vi "Convert error to warning.vi"(1 "Codes":i32[](array[numeric]), 5 "error in":errorcluster) -> (19 "error out":errorcluster)   [LabVIEW 2020]
doc: "If \"code\" is one of the code numbers given in \"Codes\", resets error status to \"no error\" and adds \"Warning: \" to \"source\"."
panel:
  # "If \"code\" is one of the code numbers given in \"Codes\", resets\nerror status to \"no error\" and adds \"Warning: \" to \"source\"."
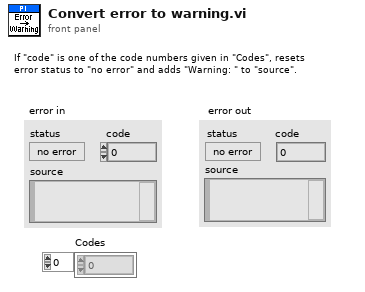
[diagram p1: front panel]
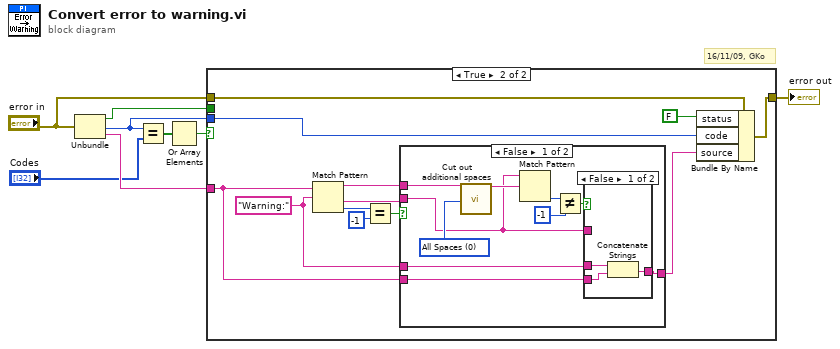
[diagram p0: block diagram]
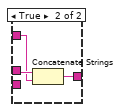
[diagram p3: hidden frame]
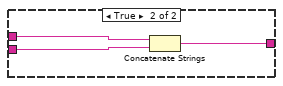
[diagram p4: hidden frame]
diagram:
  # "16/11/09, GKo"
  n1 = Unbundle("error in") -> ("status"=w7:bool, "code"=w5:i32, "source"=w6:string)
  n2 = Equal?(x=w5, y="Codes") -> (x = y?=w2:bool[])
  n3 = Or Array Elements(Boolean array=w2) -> (logical OR=w1:bool)
  n4 = case shown="True" w1 {
    tunnel: "error in" -> [w9 w21]
    tunnel: w7 -> [_ _]
    tunnel: w6 -> [_ w13]
    tunnel: w5 -> [_ w19]
    tunnel: [w9 w18] -> w4
    frame False {
    }
    frame True {
      w12 = "Warning:"
      n5 = Match Pattern(string=w13, regular expression=w12) -> (before substring=w11:string, after substring=w10:string, offset past match=w14:i32)  [unwired: 2 out]
      n6 = Equal?(x=w14, y=-1) -> (x = y?=w16:bool)
      n7 = case shown="False" w16 {
        tunnel: w13 -> [w26 w40]
        tunnel: [w28 w38] -> w15
        tunnel: w12 -> [w27 w39]
        tunnel: w11 -> [w23 _]
        tunnel: w10 -> [w22 _]
        frame False {
          w25 = u16 0 items=["All Spaces", "Only if 1st char.", "Only if last char.", "Only if near \"=\"", "Only if 1st or last char.", "Only multiple", "Really all"] ("Mode")
          n8 = call "Cut out additional spaces.vi"("String"=w23, "Mode"=w25) -> ("String out"=w24:string)  [unwired: 17 out]
          n9 = Match Pattern(string=w22, regular expression=w24) -> (offset past match=w30:i32)  [unwired: 4 out]
          n10 = Not Equal?(x=w30, y=-1) -> (x != y?=w29:bool)
          n11 = case shown="False" w29 {
            tunnel: w22 -> [_ w35]
            tunnel: [w34 w37] -> w28
            tunnel: w27 -> [w33 w36]
            tunnel: w26 -> [w32 _]
            frame False {
              n12 = Concatenate Strings(w33, w32) -> (w34:string)
            }
            frame True {
              n13 = Concatenate Strings(w36, w35) -> (w37:string)
            }
          }
        }
        frame True {
          n14 = Concatenate Strings(w39, w40) -> (w38:string)
        }
      }
      n15 = Bundle By Name(cluster=w21, "status"=FALSE, "code"=w19, "source"=w15) -> (w18:errorcluster)
    }
  }
  "error out" <- w4
